vi "F1.vi"(8 "error in (no error)":errorcluster, 9 "data":u8[](array[numeric]), 10 "function":u8, 11 "device data model in":refnum<class "Standard Data Model.lvclass">) -> (0 "error out":errorcluster, 1 "data return":u8[](array[numeric]), 2 "function return":u8, 3 "device data model out":refnum<class "Standard Data Model.lvclass">)   [LabVIEW 2020, in "SubVIs.lvlib" / "Standard Data Model.lvclass"]
doc: "Executes function code 1"
uses:
  <vilib>/Modbus/subvis/Data and Functions/Standard Data Model/Standard Data Model.lvclass
  <vilib>/Modbus/subvis/SubVIs.lvlib
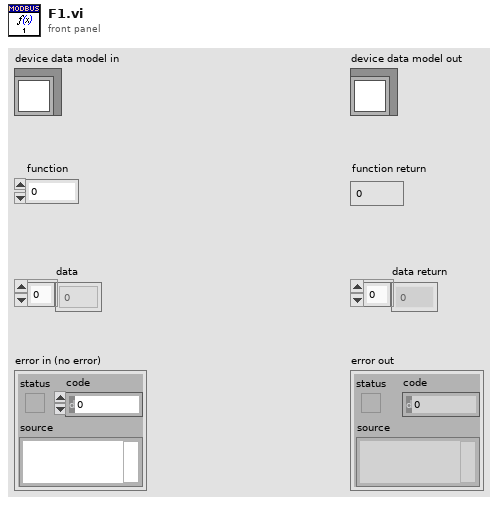
[diagram p1: front panel]
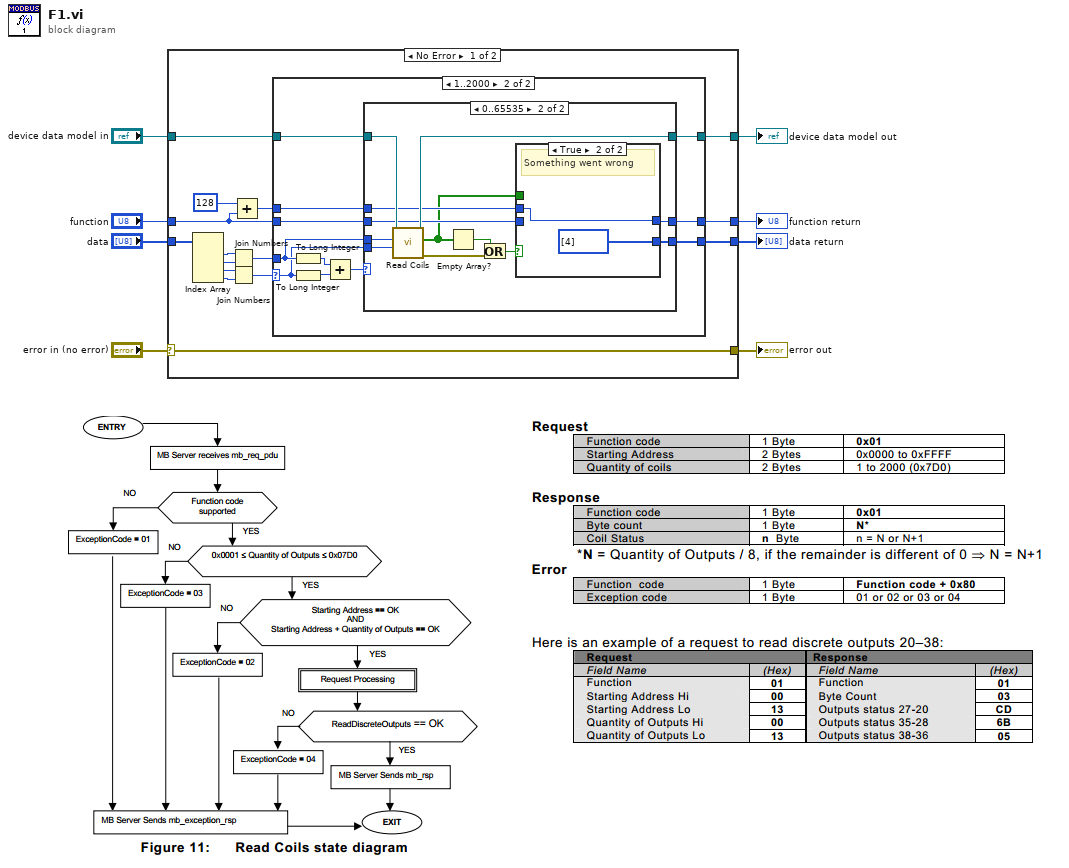
[diagram p0: block diagram]
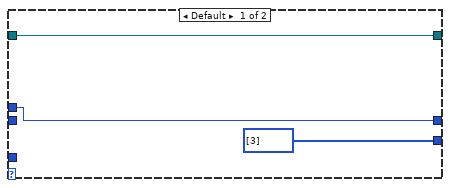
[diagram p2: hidden frame]
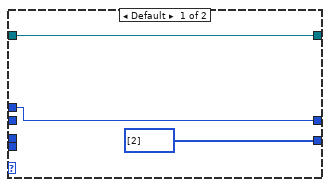
[diagram p3: hidden frame]
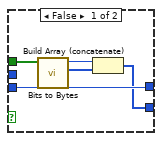
[diagram p4: hidden frame]
diagram:
  n1 = case shown="No Error" "error in (no error)" {
    selector: "error in (no error)" -> [w23 w63]
    tunnel: [w23 w63] -> w7
    tunnel: [w9 w62] -> w5
    tunnel: "device data model in" -> [w10 w62]
    tunnel: "function" -> [w16 w61]
    tunnel: "data" -> [w22 w60]
    tunnel: [w13 w61] -> w2
    tunnel: [w12 w60] -> w1
    frame No Error {
      n2 = Index Array(array=w22) -> (element #1=w20:u8, element #2=w21:u8, element #3=w19:u8, element #4=w18:u8)  [unwired: 4 in]
      n3 = Join Numbers(hi=w20, lo=w21) -> ((hi.lo)=w11:u16)
      n4 = Join Numbers(hi=w19, lo=w18) -> ((hi.lo)=w17:u16)
      n5 = Add(x=u8 128, y=w16) -> (x+y=w14:u8)
      n6 = case shown="1..2000" w17 {
        selector: w17 -> [_ w27]
        tunnel: w16 -> [_ w33]
        tunnel: w14 -> [w26 w34]
        tunnel: [w26 w32] -> w13
        tunnel: [u8[] [3] ("Data Return") w31] -> w12
        tunnel: w11 -> [_ w28]
        tunnel: w10 -> [w24 w30]
        tunnel: [w24 w29] -> w9
        frame Default {
        }
        frame 1..2000 {
          n7 = To Long Integer(number=w28) -> (32bit integer=w37:i32)
          n8 = To Long Integer(number=w27) -> (32bit integer=w36:i32)
          n9 = Add(x=w37, y=w36) -> (x+y=w35:i32)
          n10 = case shown="0..65535" w35 {
            tunnel: w34 -> [w40 w48]
            tunnel: w33 -> [_ w47]
            tunnel: [w40 w46] -> w32
            tunnel: [u8[] [2] ("Data Return") w45] -> w31
            tunnel: w30 -> [w38 w52]
            tunnel: [w38 w51] -> w29
            tunnel: w28 -> [_ w49]
            tunnel: w27 -> [_ w50]
            frame Default {
            }
            frame 0..65535 {
              n11 = call-dynamic "Read Coils.vi"("number of coils"=w50, "starting address"=w49, "device data model in"=w52) -> ("error out"=w41:errorcluster, "data"=w43:bool[], "device data model out"=w51:refnum<class "Standard Data Model.lvclass">)  [unwired: 6 in]
              n12 = Empty Array?(array=w43) -> (empty?=w42:bool)
              n13 = Or(x=w42, y=w41) -> (x .or. y?=w44:bool)
              n14 = case shown="True" w44 {
                tunnel: w43 -> [w56 _]
                tunnel: w48 -> [_ w59]
                tunnel: w47 -> [w57 _]
                tunnel: [w57 w59] -> w46
                tunnel: [w53 u8[] [4] ("Data Return")] -> w45
                frame False {
                  n15 = call <vilib>:"Bits to Bytes.vi"("bits"=w56) -> ("bytes"=w54:u8[], "count"=w55:u8)  [unwired: 9 in]
                  n16 = Build Array (concatenate)(w55, w54) -> (w53:u8[])
                }
                frame True {
                  # "Something went wrong"
                }
              }
            }
          }
        }
      }
    }
    frame Error {
    }
  }
  "error out" <- w7
  "device data model out" <- w5
  "data return" <- w1
  "function return" <- w2
